vi "Read Recordset.vi"(0 "Recordset In":refnum<k7>, 2 "Max Rows to Fetch (-1 = all)":i32=-1, 3 "error in (no error)":errorcluster) -> (4 "Field Names":string[](array[string]), 5 "Recordset Out":refnum<k7>, 6 "Data out":string[][](array[string]), 7 "Rows Returned":i32, 8 "error out":errorcluster)   [LabVIEW 2020, in "ADO Database Drivers.lvlib"]
uses:
  ADO Database Drivers.lvlib
panel:
  out "records read so far":i32
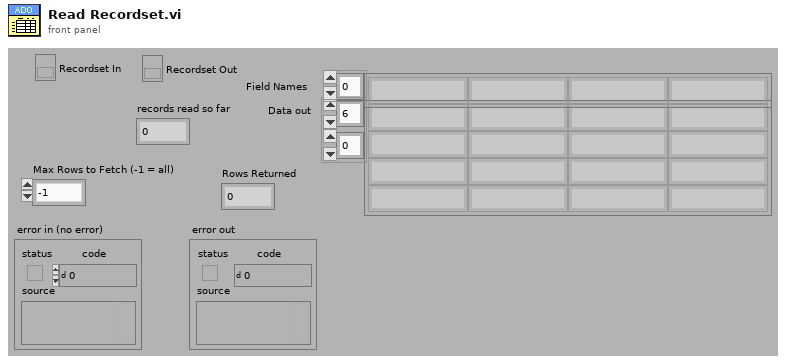
[diagram p1: front panel]
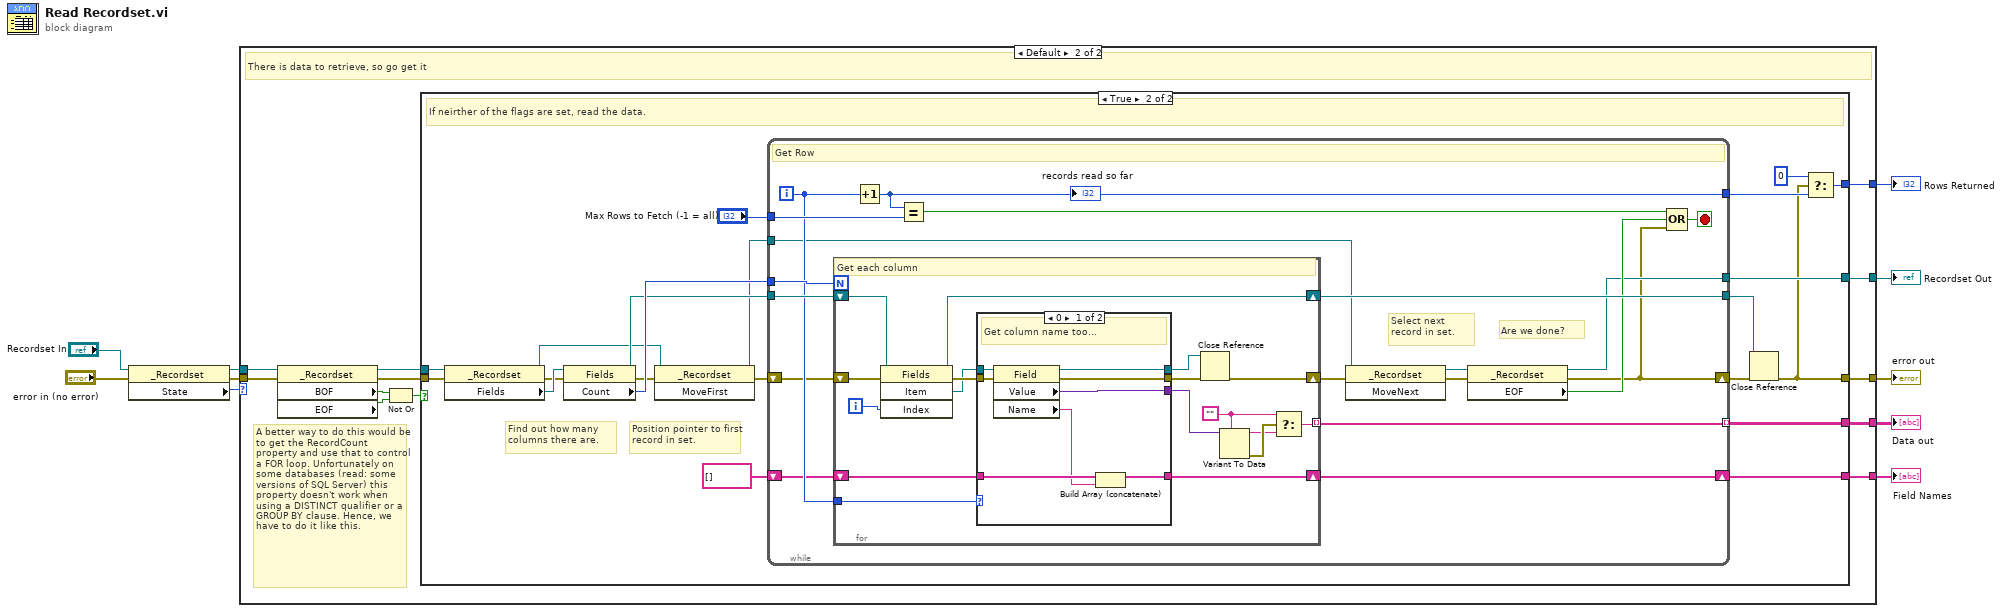
[diagram p0: block diagram]
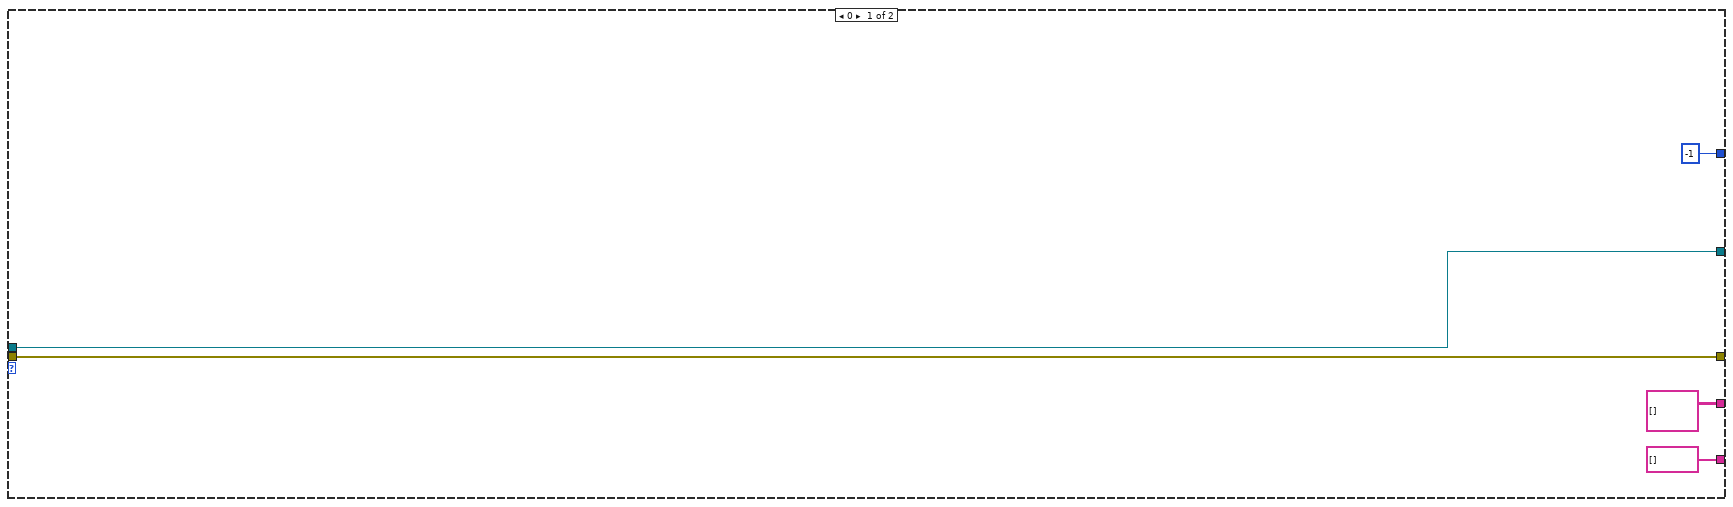
[diagram p2: hidden frame]
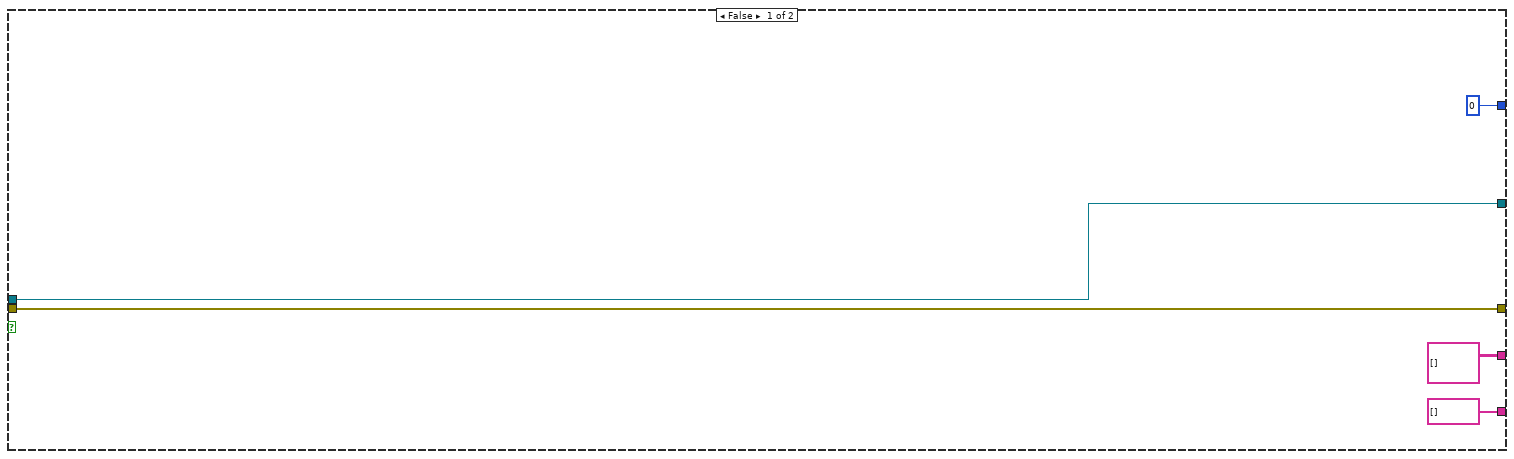
[diagram p3: hidden frame]
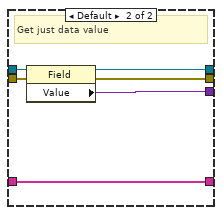
[diagram p4: hidden frame]
diagram:
  n1 = property class="_Recordset"(reference="Recordset In", error in="error in (no error)") -> (reference out=w5:refnum<k7>, error out=w3:errorcluster, "State"=w2:i32)
  n2 = case shown="Default" w2 {
    tunnel: [string[][] [] w27] -> w10
    tunnel: [w11 w26] -> w9
    tunnel: [string[] [] w25] -> w8
    tunnel: [w15 w22] -> w1
    tunnel: [-1 w21] -> w7
    tunnel: w5 -> [w11 w17]
    tunnel: w3 -> [w15 w16]
    frame 0 {
    }
    frame Default {
      # "A better way to do this would be to get the RecordCount property and use that to control a FOR loop. Unfortunately on some databases (read: some versions of SQL Server) this property doesn't work when using a DISTINCT qualifier or a GROUP BY clause. Hence, we have to do it like this."
      # "There is data to retrieve, so go get it"
      n3 = property class="_Recordset"(reference=w17, error in=w16) -> (reference out=w24:refnum<k7>, error out=w23:errorcluster, "BOF"=w20:bool, "EOF"=w18:bool)
      n4 = Not Or(1:w18, 2:w20) -> (0:w19:bool)
      n5 = case shown="True" w19 {
        tunnel: [string[][] [] w38] -> w27
        tunnel: [w32 w53] -> w26
        tunnel: [string[] [] w45] -> w25
        tunnel: w24 -> [w32 w50]
        tunnel: w23 -> [w31 w49]
        tunnel: [w31 w35] -> w22
        tunnel: [0 ("Rows Returned") w36] -> w21
        frame False {
        }
        frame True {
          # "Position pointer to first record in set."
          # "Find out how many columns there are."
          # "If neirther of the flags are set, read the data."
          n6 = property class="_Recordset"(reference=w50, error in=w49) -> (reference out=w37:refnum<k7>, error out=w51:errorcluster, "Fields"=w52:refnum<k7>)
          n7 = property class="Fields"(reference=w52, error in=w51) -> (reference out=w43:refnum<k7>, error out=w41:errorcluster, "Count"=w48:i32)
          n8 = invoke class="_Recordset" method="MoveFirst"(reference=w37, error in=w41) -> (reference out=w40:refnum<k7>, error out=w39:errorcluster)  [unwired: 1 in, 1 out]
          n9 = while {
            shift-right: [w55] -> w47
            shift-left: w39 -> [w59]
            tunnel: [w72] -> w38 mode=indexing
            tunnel: w48 -> [w71]
            tunnel: "Max Rows to Fetch (-1 = all)" -> [w67]
            tunnel: [w62] -> w46
            tunnel: w40 -> [w60]
            tunnel: [w56] -> w53
            tunnel: w43 -> [w70]
            tunnel: [w69] -> w42
            shift-right: [w64] -> w45
            shift-left: string[] [] -> [w54]
            i -> [w65]
            stop <- w68 stop-if-true
            # "Are we done?"
            # "Select next record in set."
            # "Get Row"
            n10 = for {
              N: w71 -> [_]
              shift-right: [w83] -> w61
              shift-left: w59 -> [w88]
              tunnel: [w79] -> w72 mode=indexing
              shift-right: [w84] -> w69
              shift-left: w70 -> [w85]
              tunnel: w65 -> [w76]
              shift-right: [w74] -> w64
              shift-left: w54 -> [w75]
              i -> [w73]
              w78 = ""
              # "Get each column"
              n11 = invoke class="Fields" method="Item"(reference=w85, error in=w88, "Index"=w73) -> (reference out=w84:refnum<k7>, error out=w89:errorcluster, "Item"=w77:refnum<k7>)  [unwired: 1 in, 1 out]
              n12 = case shown="0" w76 {
                tunnel: w89 -> [w97 w103]
                tunnel: [w96 w100] -> w87
                tunnel: [w95 w101] -> w86
                tunnel: [w94 w99] -> w82
                tunnel: w77 -> [w93 w102]
                tunnel: w75 -> [w92 w98]
                tunnel: [w91 w98] -> w74
                frame 0 {
                  # "Get column name too..."
                  n13 = property class="Field"(reference=w93, error in=w97) -> (reference out=w96:refnum<k7>, error out=w95:errorcluster, "Value"=w94:variant, "Name"=w90:string)
                  n14 = Build Array (concatenate)(w92, w90) -> (w91:string[])
                }
                frame Default {
                  # "Get just data value"
                  n15 = property class="Field"(reference=w102, error in=w103) -> (reference out=w100:refnum<k7>, error out=w101:errorcluster, "Value"=w99:variant)
                }
              }
              n16 = Close Reference(reference=w87, error in (no error)=w86) -> (error out=w83:errorcluster)
              n17 = Variant To Data(type=w78, Variant=w82) -> (data=w80:string, error out=w81:errorcluster)  [unwired: 1 in]
              n18 = Select(t=w78, s=w81, f=w80) -> (s? t:f=w79:string)
            }
            n19 = Increment(x=w65) -> (x+1=w62:i32)
            "records read so far" <- w62
            n20 = Equal?(x=w62, y=w67) -> (x = y?=w66:bool)
            n21 = invoke class="_Recordset" method="MoveNext"(reference=w60, error in=w61) -> (reference out=w58:refnum<k7>, error out=w57:errorcluster)  [unwired: 1 in, 1 out]
            n22 = property class="_Recordset"(reference=w58, error in=w57) -> (reference out=w56:refnum<k7>, error out=w55:errorcluster, "EOF"=w63:bool)
            n23 = Compound Arithmetic op=OR(w66, w63, w55) -> (w68:bool)
          }
          n24 = Close Reference(reference=w42, error in (no error)=w47) -> (error out=w35:errorcluster)
          n25 = Select(t=0, s=w35, f=w46) -> (s? t:f=w36:i32)
        }
      }
    }
  }
  "Data out" <- w10
  "error out" <- w1
  "Rows Returned" <- w7
  "Recordset Out" <- w9
  "Field Names" <- w8
